vi "Read Denuded.vi"(8 "error in (no error)":errorcluster, 11 "ePAS Data in":refnum<class "ePAS Data.lvclass">) -> (0 "error out":errorcluster, 2 "Denuded":bool, 3 "ePAS Data out":refnum<class "ePAS Data.lvclass">)   [LabVIEW 2014, in "ePAS Library.lvlib" / "ePAS Data.lvclass"]
uses:
  ePAS Data.lvclass
  ePAS Data.lvclass/ePAS Data.ctl
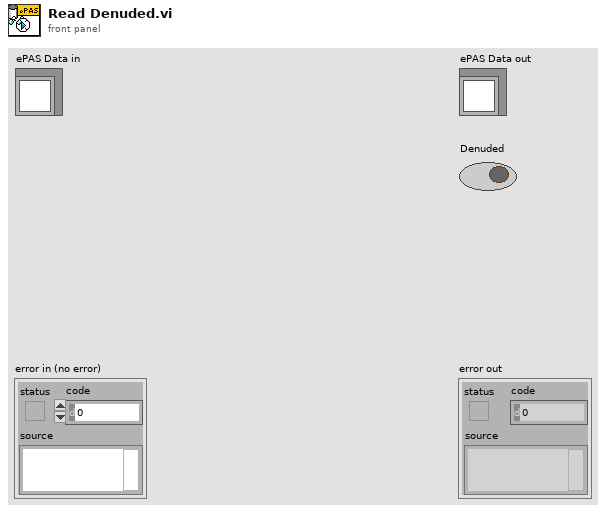
[diagram p1: front panel]
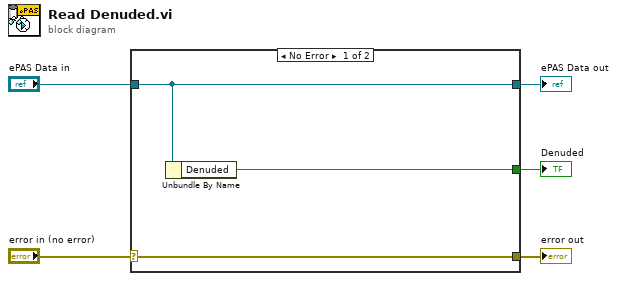
[diagram p0: block diagram]
diagram:
  n1 = case shown="No Error" "error in (no error)" {
    selector: "error in (no error)" -> [w8 w9]
    tunnel: [w8 w9] -> w4
    tunnel: [w7 w10] -> w2
    tunnel: "ePAS Data in" -> [w7 w10]
    tunnel: [w6 _] -> w1
    frame No Error {
      n2 = Unbundle By Name(w7) -> ("Denuded"=w6:bool)
    }
    frame Error {
    }
  }
  "error out" <- w4
  "ePAS Data out" <- w2
  "Denuded" <- w1
